vi "PixyCam.vi"   [LabVIEW 2017]
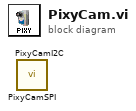
[diagram p0: block diagram]
diagram:
  n1 = call "PixyCamSPI.vi"() -> ()  [unwired: 12 in]
  n2 = call "PixyCamI2C.vi"() -> ()  [unwired: 12 in]
